vi "Initialise.vi"(8 "error in (no error)":errorcluster, 10 "Message in":refnum<class "InitialiseMessage.lvclass">, 11 "TomoConversion in":refnum<class "TomoConversion.lvclass">) -> (0 "error out":errorcluster, 3 "TomoConversion out":refnum<class "TomoConversion.lvclass">)   [LabVIEW 2012, in "TomoConversion.lvclass"]
doc: "This method is called when an initialise message is received. It mainly initialises the RabbitMQ connectivity. \n\nOverride this method when your component needs special initialisation (e.g. of software or hardware resources). In that case, don't forget to call the parent for proper implementation. If your component owns subcomponents, they count as resources, so you have to initialise them by calling their own initialise functions"
uses:
  TomoConversion.lvclass
  <vilib>/Distrio/Murmex/InitialiseMessage/InitialiseMessage.lvclass
  <vilib>/Distrio/Murmex/Murmex/Murmex.lvclass
  TomoConversion.lvclass/TomoConversion.ctl
panel:
  # "This method is called when the INTIALISE\ntrigger is sent. \n\nOverride this method when your component needs to\nrespond to this trigger. \n\nCall parent for proper implementation"
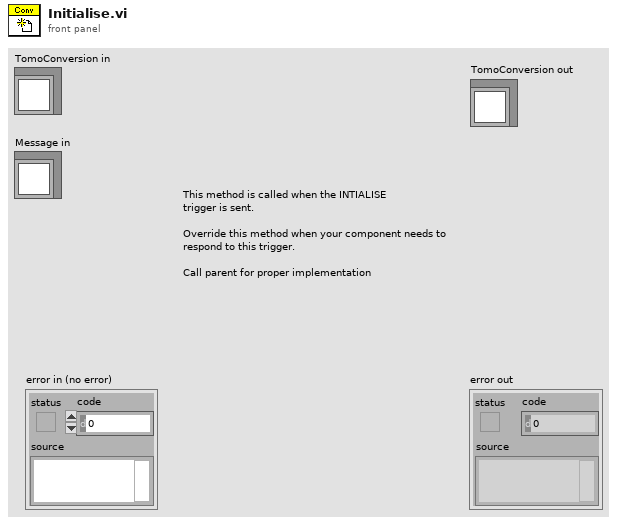
[diagram p1: front panel]
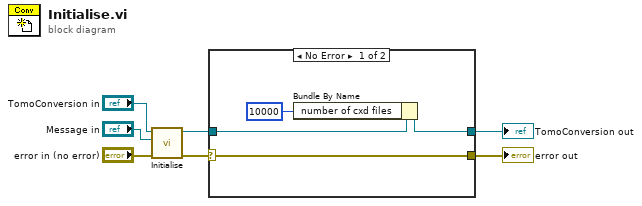
[diagram p0: block diagram]
diagram:
  n1 = call-parent "Initialise.vi"("error in (no error)"="error in (no error)", "Message in"="Message in", "Murmex in"="TomoConversion in") -> ("error out"=w2:errorcluster, "Murmex out"=w3:refnum<class "TomoConversion.lvclass">)  [unwired: 7 in]
  n2 = case shown="No Error" w2 {
    selector: w2 -> [w8 w12]
    tunnel: [w9 w13] -> w4
    tunnel: w3 -> [w11 w13]
    tunnel: [w8 w12] -> w1
    frame No Error {
      n3 = Bundle By Name(cluster=w11, "number of cxd files"=10000 ("runtime.number of cxd files")) -> (w9:refnum<class "TomoConversion.lvclass">)
    }
    frame Error {
    }
  }
  "error out" <- w1
  "TomoConversion out" <- w4
